vi "CreateLogNode.vi"(7 "DOM Document":refnum<k20>, 8 "Error In":errorcluster, 11 "Log Configuration":T1) -> (0 "Error Out":errorcluster, 3 "Log Node":refnum<k20>)   [LabVIEW 2013]
uses:
  LogConfiguration.ctl
  LogStartConfiguration.ctl
  LogStartTriggerType.ctl
  LogDigitalIOTriggerEdge.ctl
  LogRolloverConfiguration.ctl
  LogRolloverTriggerType.ctl
  LogStopConfiguration.ctl
  LogStopTriggerType.ctl
  libs/LV-Utilities/LV-Utilities.lvlib
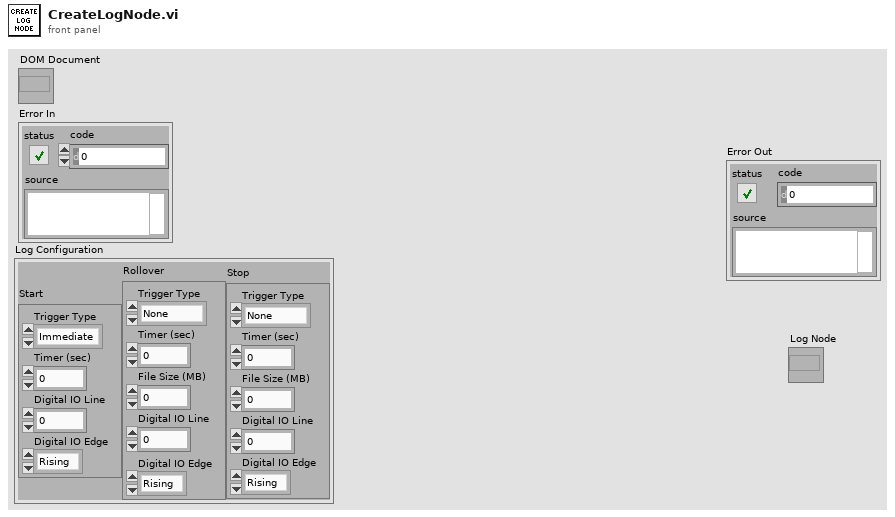
[diagram p1: front panel]
types:
  T1 = typedef "LogConfiguration.ctl" = cluster{"Start":T2, "Rollover":T5, "Stop":T7}
  T2 = typedef "LogStartConfiguration.ctl" = cluster{"Trigger Type":T3, "Timer (sec)":dbl, "Digital IO Line":u8, "Digital IO Edge":T4}
  T3 = typedef "LogStartTriggerType.ctl" = enum16{"Immediate", "User", "Timer", "Digital IO"}
  T4 = typedef "LogDigitalIOTriggerEdge.ctl" = enum16{"Rising", "Falling"}
  T5 = typedef "LogRolloverConfiguration.ctl" = cluster{"Trigger Type":T6, "Timer (sec)":dbl, "File Size (MB)":u32, "Digital IO Line":u8, "Digital IO Edge":T4}
  T6 = typedef "LogRolloverTriggerType.ctl" = enum16{"None", "Timer", "File Size", "Digital IO"}
  T7 = typedef "LogStopConfiguration.ctl" = cluster{"Trigger Type":T8, "Timer (sec)":dbl, "File Size (MB)":u32, "Digital IO Line":u8, "Digital IO Edge":T4}
  T8 = typedef "LogStopTriggerType.ctl" = enum16{"None", "User", "Timer", "File Size", "Digital IO"}
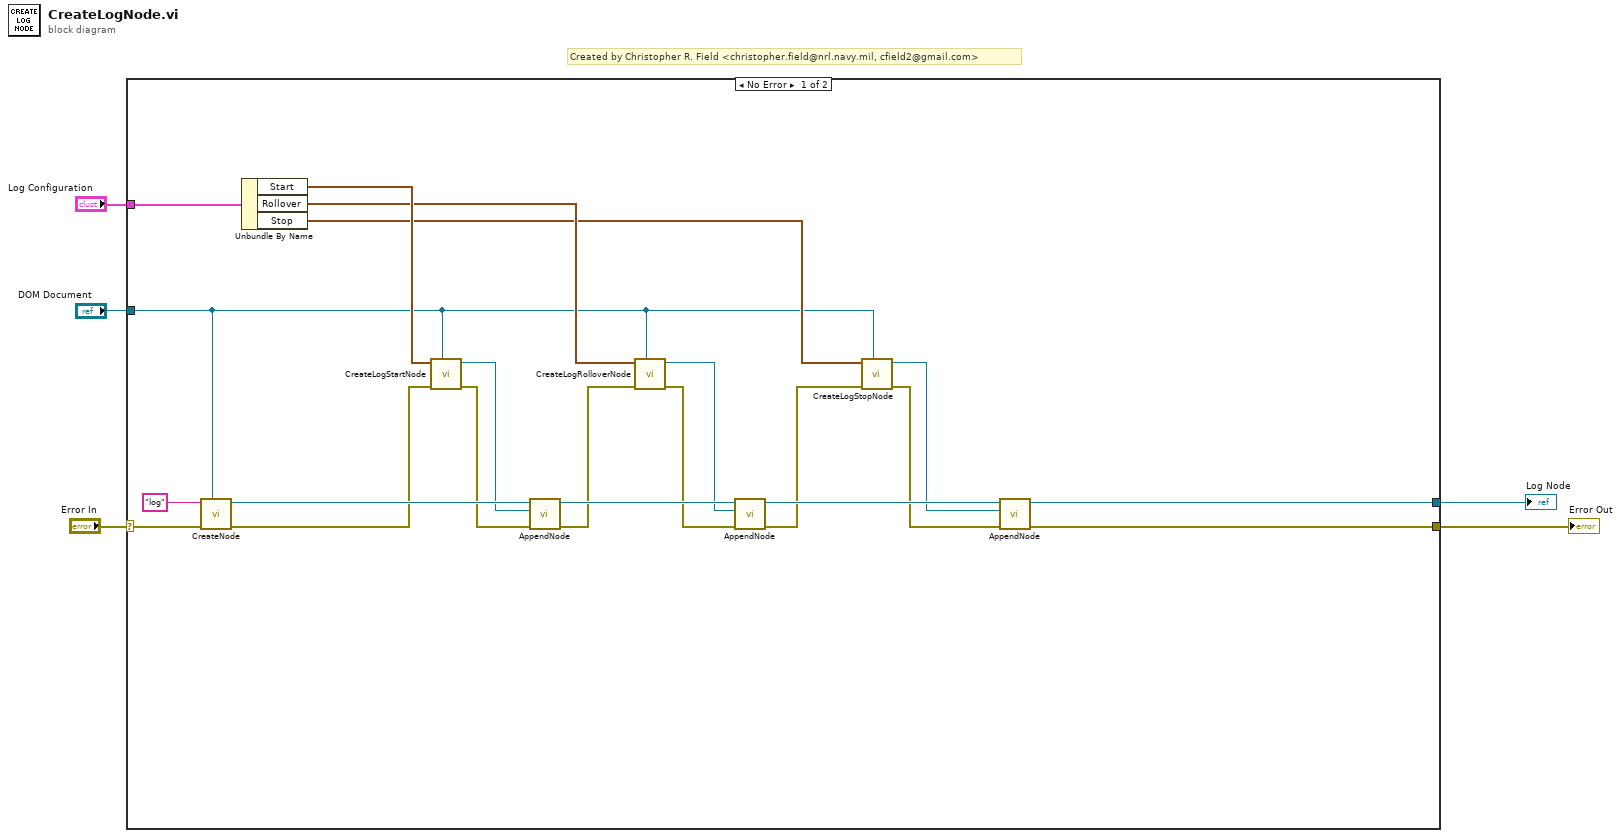
[diagram p0: block diagram]
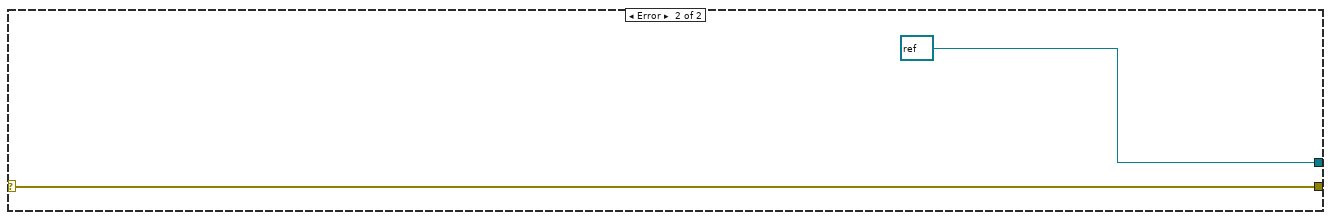
[diagram p2: hidden frame]
diagram:
  # "Created by Christopher R. Field <christopher.field@nrl.navy.mil, cfield2@gmail.com>"
  n1 = case shown="No Error" "Error In" {
    selector: "Error In" -> [w24 w28]
    tunnel: "DOM Document" -> [w9 _]
    tunnel: [w19 w28] -> w3
    tunnel: [w18 refnum<k20> refnum ("DUT Node 2")] -> w2
    tunnel: "Log Configuration" -> [w25 _]
    frame No Error {
      n2 = call "CreateNode.vi"("DOM Document"=w9, "Error In"=w24, "Tag Name"="log") -> ("Error out"=w17:errorcluster, "Node"=w22:refnum<k20>)  [unwired: 7 in]
      n3 = Unbundle By Name(w25) -> ("Start"=w26:T2, "Rollover"=w13:T5, "Stop"=w10:T7)
      n4 = call "CreateLogStartNode.vi"("DOM Document"=w9, "Error In"=w17, "Log Start Configuration"=w26) -> ("Error Out"=w16:errorcluster, "Start Node"=w15:refnum<k20>)  [unwired: 7 in]
      n5 = call "AppendNode.vi"("Error In"=w16, "Child Node"=w15, "Parent Node In"=w22) -> ("Error Out"=w14:errorcluster, "Parent Node Out"=w21:refnum<k20>)  [unwired: 7 in]
      n6 = call "CreateLogRolloverNode.vi"("DOM Document"=w9, "Error In"=w14, "Log Rollover Configuration"=w13) -> ("Error Out"=w11:errorcluster, "Rollover Node"=w12:refnum<k20>)  [unwired: 7 in]
      n7 = call "AppendNode.vi"("Error In"=w11, "Child Node"=w12, "Parent Node In"=w21) -> ("Error Out"=w8:errorcluster, "Parent Node Out"=w20:refnum<k20>)  [unwired: 7 in]
      n8 = call "CreateLogStopNode.vi"("DOM Document"=w9, "Error In"=w8, "Log Stop Configuration"=w10) -> ("Error Out"=w7:errorcluster, "Stop Node"=w6:refnum<k20>)  [unwired: 7 in]
      n9 = call "AppendNode.vi"("Error In"=w7, "Child Node"=w6, "Parent Node In"=w20) -> ("Error Out"=w19:errorcluster, "Parent Node Out"=w18:refnum<k20>)  [unwired: 7 in]
    }
    frame Error {
    }
  }
  "Error Out" <- w3
  "Log Node" <- w2
